vi "Test_Int.vi"(8 "error in (no error)":errorcluster, 10 "Parameters":string, 11 "reference in":refnum<class "Test_Sim.lvclass">) -> (0 "error out":errorcluster, 2 "Result":i32, 3 "reference in":refnum<class "Test_Sim.lvclass">)   [LabVIEW 2020, in "Test_Sim.lvlib" / "Test_Sim.lvclass"]
uses:
  Test_Sim.lvclass
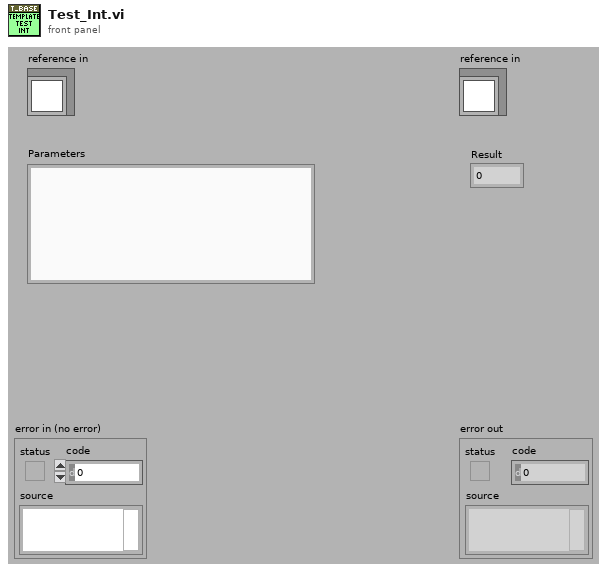
[diagram p1: front panel]
types:
  T1 = typedef "Test_Sim.lvlib/Test_Sim.lvclass/ObjectAttributes.ctl" = cluster{"Config":T2}
  T2 = typedef "Test_Sim.lvlib/Test_Sim.lvclass/Config.ctl" = cluster{"_default":string}
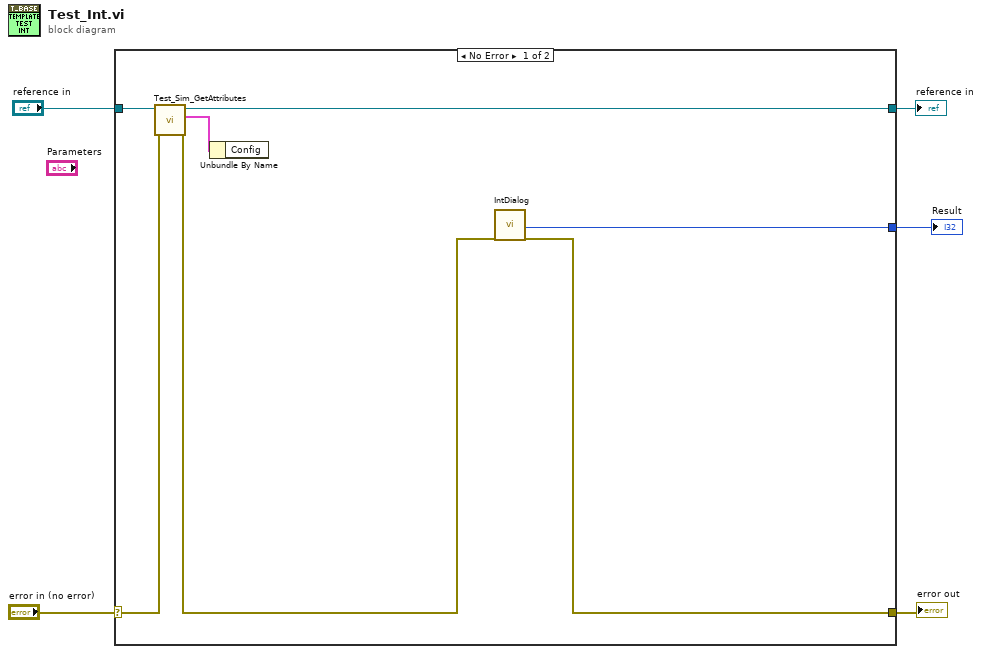
[diagram p0: block diagram]
diagram:
  n1 = case shown="No Error" "error in (no error)" {
    selector: "error in (no error)" -> [w12 w14]
    tunnel: [w6 w14] -> w4
    tunnel: [w9 w13] -> w2
    tunnel: "reference in" -> [w10 w13]
    tunnel: [w8 _] -> w1
    frame No Error {
      n2 = call "Test_Sim_GetAttributes.vi"("error in (no error)"=w12, "reference in"=w10) -> ("error out"=w7:errorcluster, "Data"=w11:T1, "reference out"=w9:refnum<class "Test_Sim.lvclass">)  [unwired: 6 in, 1 out]
      n3 = Unbundle By Name(w11) -> ()  [unwired: 1 out]
      n4 = call "IntDialog.vi"("error in (no error)"=w7) -> ("Value"=w8:i32, "error out"=w6:errorcluster)  [unwired: 16 in, 1 out]
    }
    frame Error {
    }
  }
  "error out" <- w4
  "reference in" <- w2
  "Result" <- w1
